vi "Configure Sequencer List Dwell Time.vi"(7 "Dwell Time (1.0E-3)":dbl=0.001 format="%^.3e", 8 "error in (no error)":errorcluster, 9 "Index (0)":i32, 10 "Instance (1)":i32=1, 11 "VISA resource name":refnum<visa-resource-name>) -> (0 "error out":errorcluster, 3 "VISA resource name out":refnum<visa-resource-name>)   [LabVIEW 2015, in "Rohde&Schwarz CMXP GPRF.lvlib"]
doc: "Defines the dwell time for the sequencer list entry with the selected Index.\n\nAttribute:\nRSCMXPGPRF_ATTR_SEQUENCER_LIST_DWELL_TIME\n\nRemote-control command:\nSOURce:GPRF:GEN<i>:SEQuencer:LIST:DTIMe"
uses:
  <instrlib>/Rohde&Schwarz CMXP GPRF/Rohde&Schwarz CMXP GPRF.lvlib
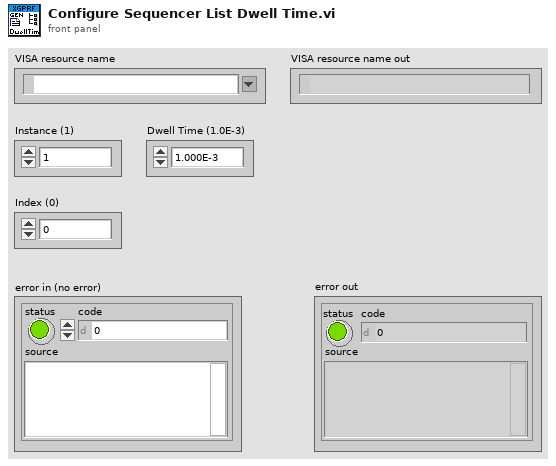
[diagram p1: front panel]
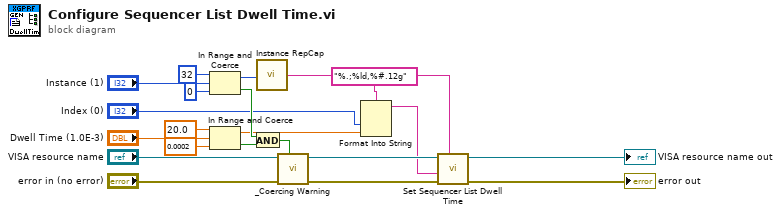
[diagram p0: block diagram]
diagram:
  n1 = In Range and Coerce(upper limit=32, x="Instance (1)", lower limit=0) -> (coerced(x)=w6:i32, In Range?=w17:bool)
  n2 = In Range and Coerce(upper limit=20.0, x="Dwell Time (1.0E-3)", lower limit=0.0002) -> (coerced(x)=w2:dbl, In Range?=w11:bool)
  n3 = And(x=w17, y=w11) -> (x .and. y?=w16:bool)
  n4 = call <instrlib>:"Instance RepCap.vi"("Instance in"=w6) -> ("Instance out"=w5:string)
  n5 = call <instrlib>:"_Coercing Warning.vi"("In Range?"=w16, "error in (no error)"="error in (no error)", "VISA resource name"="VISA resource name") -> ("error out"=w10:errorcluster, "VISA resource name out"=w9:refnum<visa-resource-name>)  [unwired: 7 in]
  n6 = Format Into String(format string="%.;%ld,%#.12g", "Index (0)", w2) -> (resulting string=w1:string)  [unwired: 2 in, 1 out]
  n7 = call "Set Sequencer List Dwell Time"("Repeated Capabilities"=w5, "error in (no error)"=w10, "Sequencer List Dwell Time ()"=w1, "instrument handle"=w9) -> ("error out"=→"error out":errorcluster, "instrument handle out"=→"VISA resource name out":refnum<visa-resource-name>)  [unwired: 6 in]
